vi "shutterStatusToAceFormat.vi"(8 "error in (no error)":errorcluster, 10 "lineStatus":string, 11 "DomeCommunicator in":refnum<class "ATDomeCommunicator.lvclass">) -> (0 "error out":errorcluster, 1 "openingPercentage":T1 min=0.0 max=100.0, 2 "shutterStatus":T2, 3 "DomeCommunicator out":refnum<class "ATDomeCommunicator.lvclass">)   [LabVIEW 2016, in "ATDomeCommunicator.lvclass"]
uses:
  ATDomeCommunicator.lvclass
  ComTypedefs/openingStates.ctl
  IDome/domeTypedefs/openingPercentage.ctl
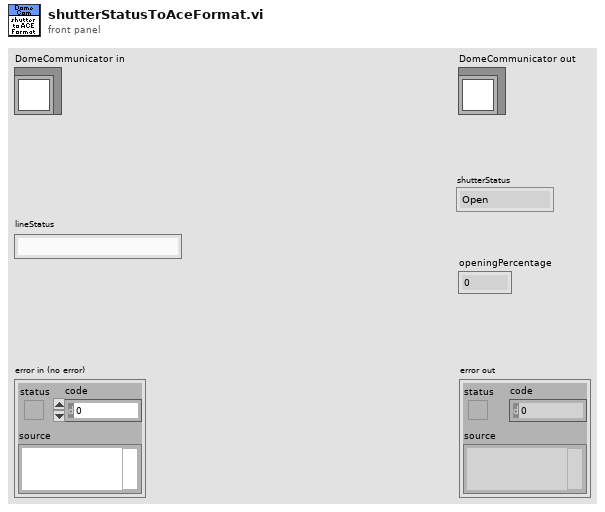
[diagram p1: front panel]
types:
  T1 = typedef "openingPercentage.ctl" = dbl
  T2 = typedef "openingStates.ctl" = enum16{"Open", "Shut", "Ajar"}
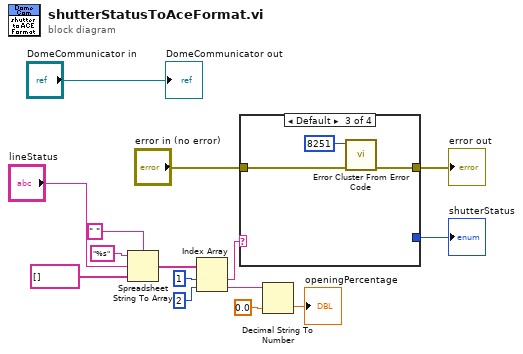
[diagram p0: block diagram]
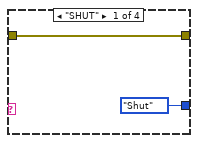
[diagram p2: hidden frame]
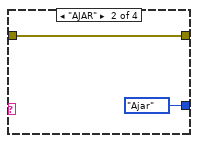
[diagram p3: hidden frame]
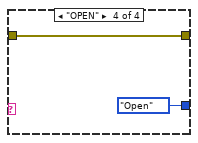
[diagram p4: hidden frame]
diagram:
  n1 = Spreadsheet String To Array(delimiter (Tab)=" ", format string="%s", spreadsheet string="lineStatus", array type (2D Dbl)=string[] []) -> (array=w10:string[])
  n2 = Index Array(array=w10, index #1=1 ("index"), index #2=2 ("index")) -> (element #1=w4:string, element #2=w7:string)
  n3 = case shown="Default" w4 {
    tunnel: "error in (no error)" -> [w17 w18 w21 w23]
    tunnel: [openingStates."Shut" ("openingState") openingStates."Ajar" ("openingState") _ openingStates."Open" ("openingState")] -> w2
    tunnel: [w17 w18 w22 w23] -> w1
    frame "SHUT" {
    }
    frame "AJAR" {
    }
    frame Default {
      n4 = call <vilib>:"Error Cluster From Error Code.vi"("error in (no error)"=w21, "error code (0)"=8251) -> ("error out"=w22:errorcluster)  [unwired: 7 in]
    }
    frame "OPEN" {
    }
  }
  "error out" <- w1
  "shutterStatus" <- w2
  n5 = Decimal String To Number(string=w7, default (0L)=T1 0.0 ("openingPercentage")) -> (number=→"openingPercentage":dbl)  [unwired: 1 in, 1 out]
  "DomeCommunicator out" <- "DomeCommunicator in"
